vi "Format WFM Data for File.vi"(7 "DAQmx Task Name":refnum<k21>, 8 "error in (no error)":errorcluster, 11 "Data Setup":refnum<vi>) -> (0 "error IO":errorcluster, 2 "Headers":string[](array[string]), 3 "Header":string)   [LabVIEW 2017]
uses:
  <resource>/objmgr/daqmx.rc
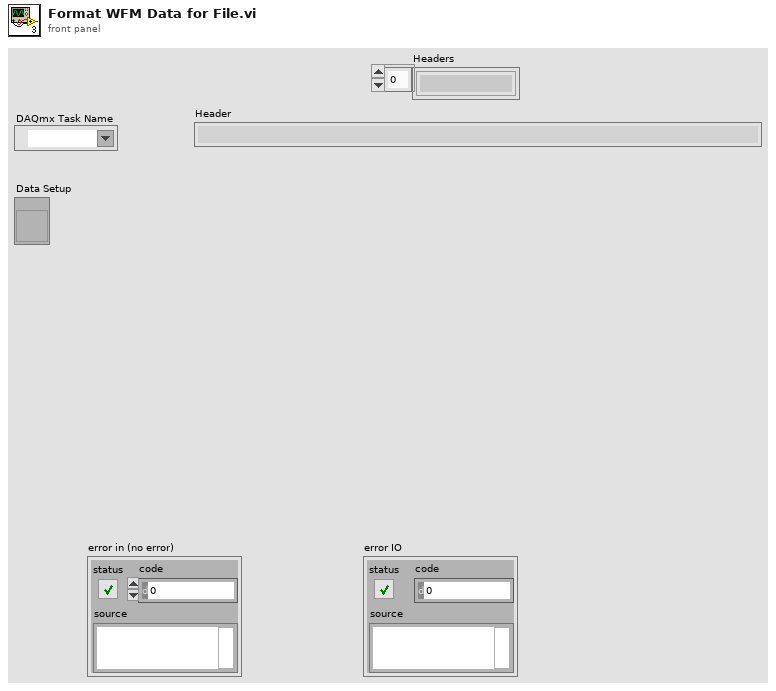
[diagram p1: front panel]
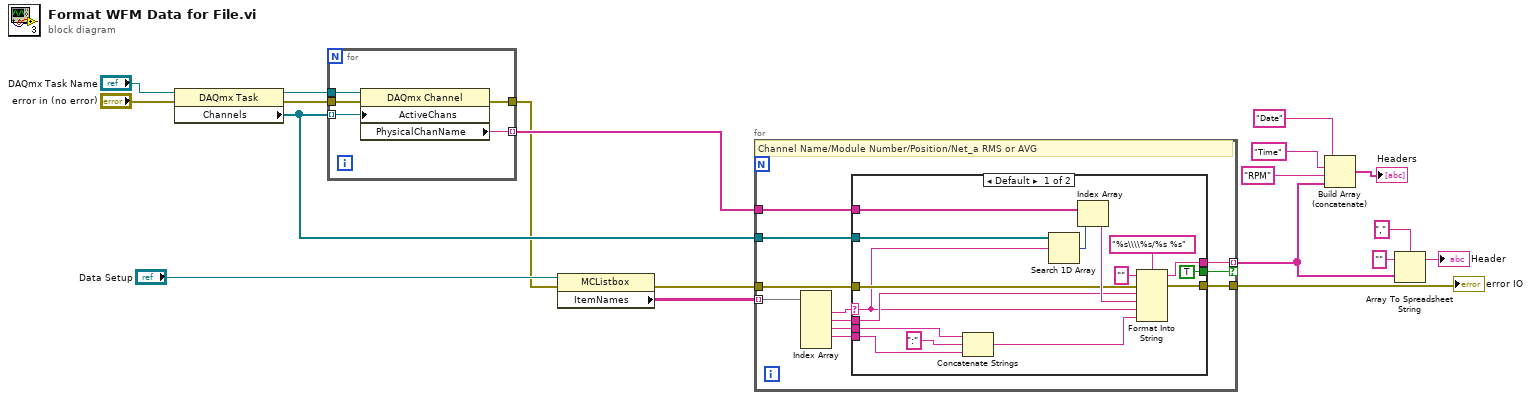
[diagram p0: block diagram]
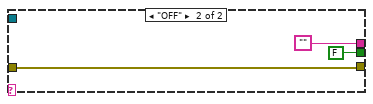
[diagram p2: hidden frame]
diagram:
  n1 = property class="DAQmx Task"(reference="DAQmx Task Name", error in="error in (no error)") -> (reference out=w18:refnum<k21>, error out=w17:errorcluster, "Channels"=w14:refnum<k21>[])
  n2 = for {
    tunnel: w18 -> [w24]
    tunnel: w14 -> [w22] mode=indexing
    tunnel: w17 -> [w23]
    tunnel: [w21] -> w15 mode=indexing
    tunnel: [w20] -> w11
    n3 = property class="DAQmx Channel"(reference=w24, error in=w23, "ActiveChans"=w22) -> (error out=w20:errorcluster, "PhysicalChanName"=w21:tag)  [unwired: 1 out]
  }
  n4 = property on="Property Node" class="MCListbox"(reference="Data Setup", error in=w11) -> (error out=w10:errorcluster, "ItemNames"=w13:string[][])  [unwired: 1 out]
  n5 = for {
    tunnel: w13 -> [w35] mode=indexing
    tunnel: w14 -> [w34]
    tunnel: w15 -> [w33]
    tunnel: [w31] -> w7 mode=indexing if=w25
    tunnel: w10 -> [w30]
    tunnel: [w29] -> w9
    # "Channel Name/Module Number/Position/Net_a RMS or AVG"
    n6 = Index Array(array=w35) -> (element #1=w26:string, element #2=w32:string, element #3=w28:string, element #4=w27:string)  [unwired: 5 in, 1 out]
    n7 = case shown="Default" w26 {
      selector: w26 -> [w37 _]
      tunnel: w34 -> [w51 _]
      tunnel: w33 -> [w50 _]
      tunnel: w32 -> [w47 _]
      tunnel: [w45 ""] -> w31
      tunnel: w30 -> [w43 w54]
      tunnel: [w42 w54] -> w29
      tunnel: w28 -> [w41 _]
      tunnel: w27 -> [w39 _]
      tunnel: [TRUE FALSE] -> w25
      frame Default {
        n8 = Concatenate Strings(w41, ":", w39) -> (w40:string)
        n9 = Search 1D Array(1D array=w51, element=w37) -> (index of element=w46:i32)  [unwired: 1 in]
        n10 = Index Array(array=w50, index=w46) -> (element=w48:tag)
        n11 = Format Into String(format string="%s\\\\%s/%s %s", initial string="", error in=w43, w47, w48, w37, w40) -> (resulting string=w45:string, error out=w42:errorcluster)
      }
      frame "OFF" {
      }
    }
  }
  "error IO" <- w9
  n12 = Build Array (concatenate)("Date" ("format string"), "Time" ("format string"), "RPM" ("element"), w7) -> (→"Headers":string[])
  n13 = Array To Spreadsheet String(delimiter (Tab)=",", array=w7, 3:"" ("format string")) -> (spreadsheet string=→"Header":string)
